vi "Create XRay Table.vi"(8 "error in (no error)":errorcluster, 11 "XRay Table in":refnum<class "XRay Table.lvclass">) -> (0 "error out":errorcluster, 3 "XRay Table out":refnum<class "XRay Table.lvclass">)   [LabVIEW 2026, in "XRay Table.lvclass"]
uses:
  XRay Table.lvclass
  XRay Table.lvclass/XRay Table.ctl
  <vilib>/picture/3D Picture Control/Object/Create Object (drawable).vi
  <vilib>/picture/3D Picture Control/NI_3D Picture Control.lvlib
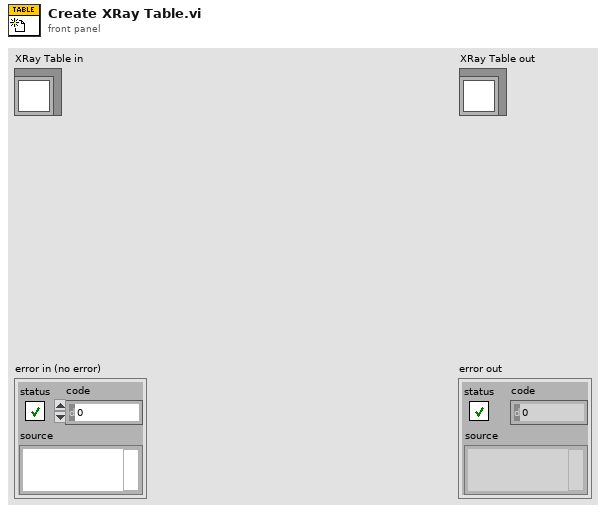
[diagram p1: front panel]
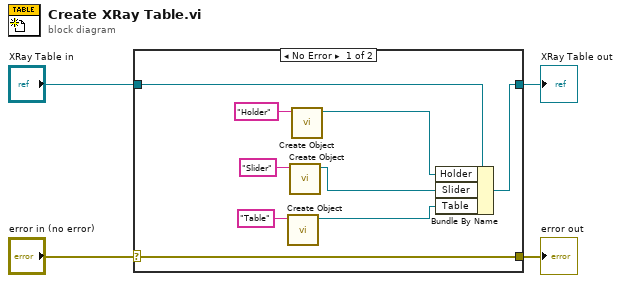
[diagram p0: block diagram]
diagram:
  n1 = case shown="No Error" "error in (no error)" {
    selector: "error in (no error)" -> [w13 w14]
    tunnel: [w13 w14] -> w3
    tunnel: [w11 w15] -> w1
    tunnel: "XRay Table in" -> [w12 w15]
    frame No Error {
      n2 = call-poly <vilib>:"Create Object.vi"("Name"="Table") -> ("Scene:New Object"=w5:refnum<vi>)  [unwired: 9 in, 1 out]
      n3 = call-poly <vilib>:"Create Object.vi"("Name"="Slider") -> ("Scene:New Object"=w6:refnum<vi>)  [unwired: 9 in, 1 out]
      n4 = call-poly <vilib>:"Create Object.vi"("Name"="Holder") -> ("Scene:New Object"=w7:refnum<vi>)  [unwired: 9 in, 1 out]
      n5 = Bundle By Name(cluster=w12, "Holder"=w7, "Slider"=w6, "Table"=w5) -> (w11:refnum<class "XRay Table.lvclass">)
    }
    frame Error {
    }
  }
  "error out" <- w3
  "XRay Table out" <- w1
